vi "3color creation-cluster-2.vi"(4 "color":T1(array[cluster]) {"min" step=0.01 format="%_2f"; "max" step=0.1 format="%_3f"}, 5 "Array 4":bool[](array[boolean])=[TRUE, TRUE, TRUE], 7 "Array 3":dbl[][](array[numeric])=array90x160[14400 elements], 8 "Array 2":dbl[][](array[numeric])=array90x160[14400 elements], 9 "Array":dbl[][](array[numeric])=array90x160[14400 elements]) -> (0 "new picture":picture, 1 "ch3":picture, 2 "ch2":picture, 3 "ch1":picture)   [LabVIEW 2018]
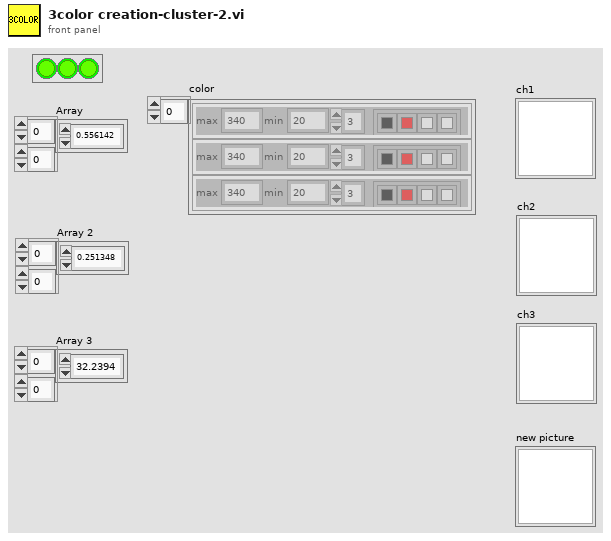
[diagram p1: front panel]
types:
  T1 = cluster{"color array":u32[], "num of colors":i32, "max":dbl, "min":dbl}[]
  T2 = cluster{"color array":u32[], "num of colors":i32, "max":dbl, "min":dbl}
  T3 = typedef "imagedata.ctl" = cluster{"image type":i32, "image depth":i32, "image":u8[], "mask":u8[], "colors":u32[], "Rectangle":cluster{"left":i16, "top":i16, "right":i16, "bottom":i16}}
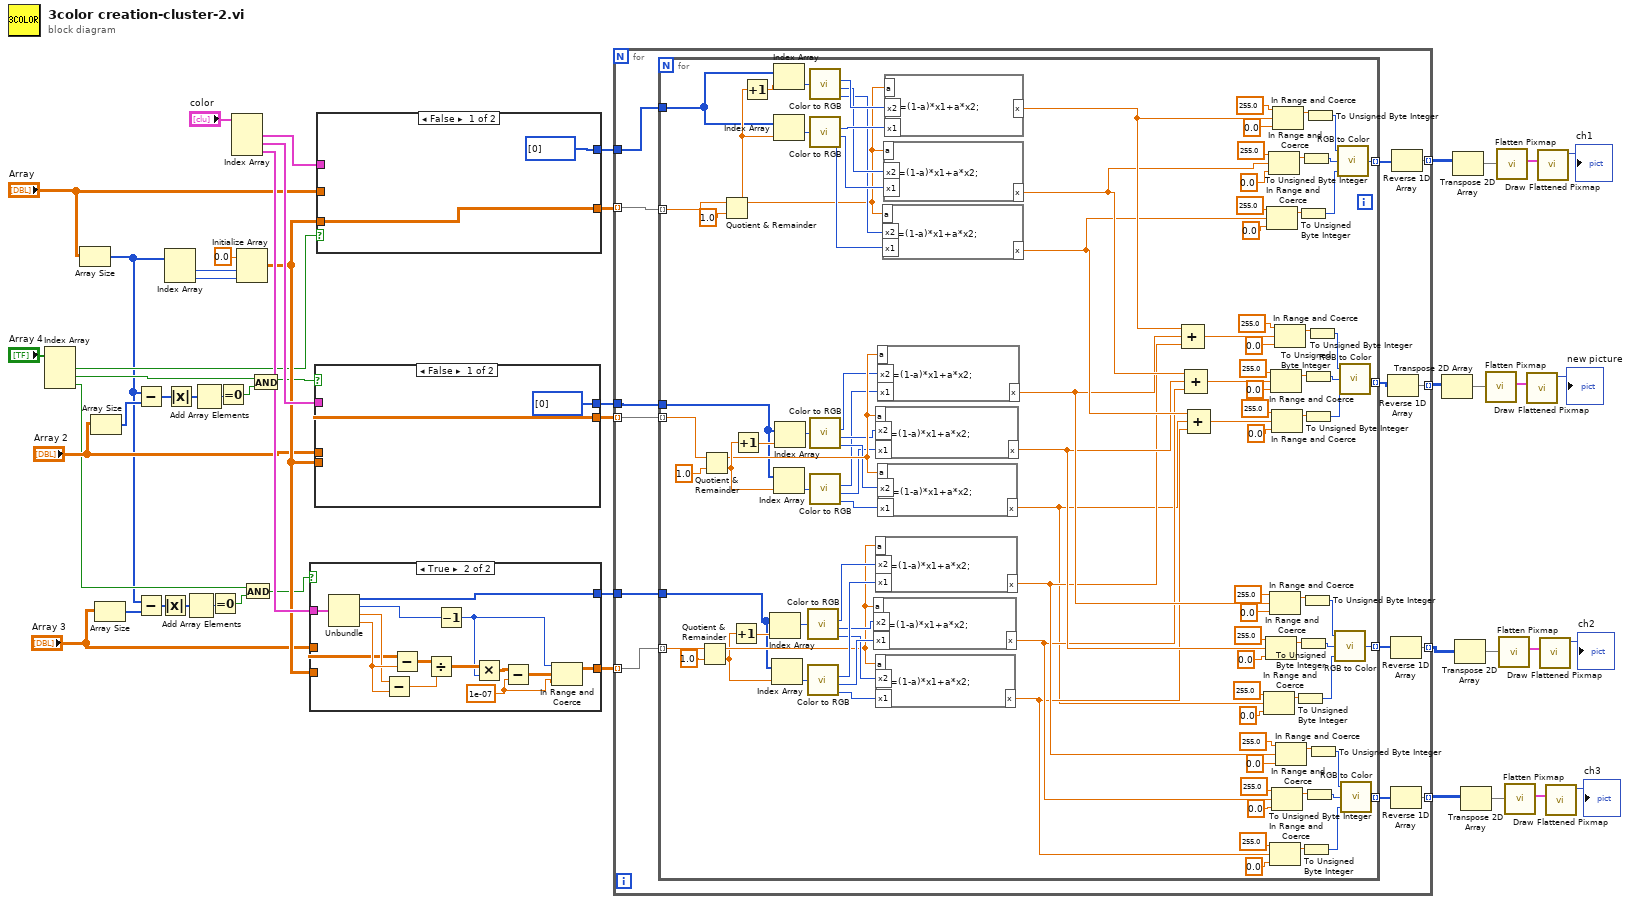
[diagram p0: block diagram]
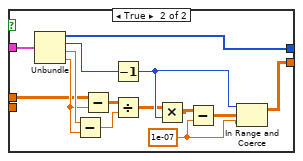
[diagram p2: hidden frame]
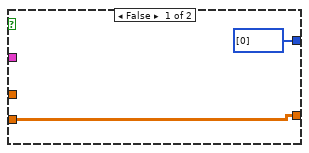
[diagram p3: hidden frame]
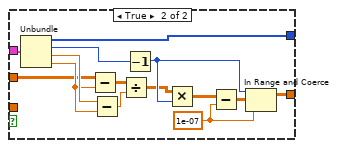
[diagram p4: hidden frame]
diagram:
  n1 = Index Array(array="Array 4") -> (element #1=w19:bool, element #2=w18:bool, element #3=w6:bool)  [unwired: 3 in]
  n2 = Array Size(array="Array") -> (size(s)=w4:i32[])
  n3 = Array Size(array="Array 2") -> (size(s)=w14:i32[])
  n4 = Array Size(array="Array 3") -> (size(s)=w7:i32[])
  n5 = Subtract(x=w4, y=w14) -> (x-y=w13:i32[])
  n6 = Subtract(x=w4, y=w7) -> (x-y=w8:i32[])
  n7 = Absolute Value(x=w8) -> (abs(x)=w2:i32[])
  n8 = Index Array(array=w4) -> (element #1=w22:i32, element #2=w23:i32)  [unwired: 2 in]
  n9 = Absolute Value(x=w13) -> (abs(x)=w1:i32[])
  n10 = Add Array Elements(numeric array=w2) -> (sum=w9:i32)
  n11 = Add Array Elements(numeric array=w1) -> (sum=w12:i32)
  n12 = Equal To 0?(x=w9) -> (x = 0?=w10:bool)
  n13 = Equal To 0?(x=w12) -> (x = 0?=w11:bool)
  n14 = Index Array(array="color") -> (element #1=w27:T2, element #2=w26:T2, element #3=w25:T2)  [unwired: 3 in]
  n15 = Initialize Array(0.0 ("element"), w22, w23) -> (w20:dbl[][])
  n16 = And(x=w6, y=w10) -> (x .and. y?=w5:bool)
  n17 = And(x=w18, y=w11) -> (x .and. y?=w15:bool)
  n18 = case shown="True" w5 {
    tunnel: [u32[] [0] ("color array") w56] -> w43
    tunnel: [w52 w55] -> w42
    tunnel: w25 -> [_ w54]
    tunnel: "Array 3" -> [_ w53]
    tunnel: w20 -> [w52 _]
    frame False {
    }
    frame True {
      w59 = 1e-07
      n19 = Unbundle(w54) -> ("color array"=w56:u32[], "num of colors"=w61:i32, "max"=w64:dbl, "min"=w65:dbl)
      n20 = Subtract(x=w64, y=w65) -> (x-y=w62:dbl)
      n21 = Subtract(x=w53, y=w65) -> (x-y=w63:dbl[][])
      n22 = Divide(x=w63, y=w62) -> (x/y=w66:dbl[][])
      n23 = Decrement(x=w61) -> (x-1=w57:i32)
      n24 = Multiply(x=w66, y=w57) -> (x*y=w58:dbl[][])
      n25 = Subtract(x=w58, y=w59) -> (x-y=w60:dbl[][])
      n26 = In Range and Coerce(upper limit=w57, x=w60, lower limit=w59) -> (coerced(x)=w55:dbl[][])  [unwired: 1 out]
    }
  }
  n27 = case shown="False" w15 {
    tunnel: [w68 w82] -> w50
    tunnel: [u32[] [0] ("color array") w81] -> w44
    tunnel: w26 -> [_ w80]
    tunnel: "Array 2" -> [_ w69]
    tunnel: w20 -> [w68 _]
    frame False {
    }
    frame True {
      w77 = 1e-07
      n28 = Unbundle(w80) -> ("color array"=w81:u32[], "num of colors"=w75:i32, "max"=w72:dbl, "min"=w71:dbl)
      n29 = Subtract(x=w72, y=w71) -> (x-y=w74:dbl)
      n30 = Subtract(x=w69, y=w71) -> (x-y=w73:dbl[][])
      n31 = Decrement(x=w75) -> (x-1=w79:i32)
      n32 = Divide(x=w73, y=w74) -> (x/y=w70:dbl[][])
      n33 = Multiply(x=w70, y=w79) -> (x*y=w78:dbl[][])
      n34 = Subtract(x=w78, y=w77) -> (x-y=w76:dbl[][])
      n35 = In Range and Coerce(upper limit=w79, x=w76, lower limit=w77) -> (coerced(x)=w82:dbl[][])  [unwired: 1 out]
    }
  }
  n36 = case shown="False" w19 {
    tunnel: [w84 w96] -> w48
    tunnel: [u32[] [0] ("color array") w93] -> w45
    tunnel: w27 -> [_ w86]
    tunnel: "Array" -> [_ w85]
    tunnel: w20 -> [w84 _]
    frame False {
    }
    frame True {
      w95 = 1e-07
      n37 = Unbundle(w86) -> ("color array"=w93:u32[], "num of colors"=w92:i32, "max"=w91:dbl, "min"=w90:dbl)
      n38 = Subtract(x=w85, y=w90) -> (x-y=w89:dbl[][])
      n39 = Subtract(x=w91, y=w90) -> (x-y=w88:dbl)
      n40 = Divide(x=w89, y=w88) -> (x/y=w87:dbl[][])
      n41 = Decrement(x=w92) -> (x-1=w98:i32)
      n42 = Multiply(x=w87, y=w98) -> (x*y=w97:dbl[][])
      n43 = Subtract(x=w97, y=w95) -> (x-y=w94:dbl[][])
      n44 = In Range and Coerce(upper limit=w98, x=w94, lower limit=w95) -> (coerced(x)=w96:dbl[][])  [unwired: 1 out]
    }
  }
  n45 = for {
    tunnel: w48 -> [w112] mode=indexing
    tunnel: w45 -> [w111]
    tunnel: w50 -> [w110] mode=indexing
    tunnel: [w107] -> w46 mode=indexing
    tunnel: w44 -> [w108]
    tunnel: w43 -> [w106]
    tunnel: w42 -> [w105] mode=indexing
    tunnel: [w103] -> w29 mode=indexing
    tunnel: [w101] -> w30 mode=indexing
    tunnel: [w99] -> w31 mode=indexing
    n46 = for {
      tunnel: w112 -> [w114] mode=indexing
      tunnel: w111 -> [w194]
      tunnel: w110 -> [w113] mode=indexing
      tunnel: [w193] -> w109 mode=indexing
      tunnel: w108 -> [w192]
      tunnel: w106 -> [w164]
      tunnel: w105 -> [w163] mode=indexing
      tunnel: [w124] -> w100 mode=indexing
      tunnel: [w123] -> w102 mode=indexing
      tunnel: [w122] -> w104 mode=indexing
      n47 = Quotient & Remainder(x=w163, y=1.0) -> (x-y*floor(x/y)=w166:dbl, floor(x/y)=w165:dbl)
      n48 = Quotient & Remainder(x=w113, y=1.0) -> (x-y*floor(x/y)=w205:dbl, floor(x/y)=w206:dbl)
      n49 = Quotient & Remainder(x=w114, y=1.0) -> (x-y*floor(x/y)=w208:dbl, floor(x/y)=w207:dbl)
      n50 = Increment(x=w165) -> (x+1=w175:dbl)
      n51 = Increment(x=w206) -> (x+1=w196:dbl)
      n52 = Increment(x=w207) -> (x+1=w217:dbl)
      n53 = Index Array(array=w164, index=w175) -> (element=w174:u32)
      n54 = Index Array(array=w164, index=w165) -> (element=w173:u32)
      n55 = Index Array(array=w194, index=w217) -> (element=w216:u32)
      n56 = Index Array(array=w194, index=w207) -> (element=w215:u32)
      n57 = Index Array(array=w192, index=w206) -> (element=w198:u32)
      n58 = Index Array(array=w192, index=w196) -> (element=w197:u32)
      n59 = call <vilib>:"Color to RGB.vi"("Color"=w174) -> ("R"=w171:u8, "G"=w169:u8, "B"=w167:u8)  [unwired: 1 out]
      n60 = call <vilib>:"Color to RGB.vi"("Color"=w173) -> ("R"=w172:u8, "G"=w170:u8, "B"=w168:u8)  [unwired: 1 out]
      n61 = call <vilib>:"Color to RGB.vi"("Color"=w216) -> ("R"=w213:u8, "G"=w211:u8, "B"=w209:u8)  [unwired: 1 out]
      n62 = call <vilib>:"Color to RGB.vi"("Color"=w215) -> ("R"=w214:u8, "G"=w212:u8, "B"=w210:u8)  [unwired: 1 out]
      n63 = call <vilib>:"Color to RGB.vi"("Color"=w197) -> ("R"=w200:u8, "G"=w202:u8, "B"=w204:u8)  [unwired: 1 out]
      n64 = call <vilib>:"Color to RGB.vi"("Color"=w198) -> ("R"=w199:u8, "G"=w201:u8, "B"=w203:u8)  [unwired: 1 out]
      n65 = formula code="x=(1-a)*x1+a*x2;"("a"=w166, "x2"=w169, "x1"=w170) -> ("x"=w126:dbl)
      n66 = formula code="x=(1-a)*x1+a*x2;"("a"=w205, "x2"=w202, "x1"=w201) -> ("x"=w128:dbl)
      n67 = formula code="x=(1-a)*x1+a*x2;"("a"=w166, "x2"=w171, "x1"=w172) -> ("x"=w127:dbl)
      n68 = formula code="x=(1-a)*x1+a*x2;"("a"=w166, "x2"=w167, "x1"=w168) -> ("x"=w125:dbl)
      n69 = formula code="x=(1-a)*x1+a*x2;"("a"=w205, "x2"=w200, "x1"=w199) -> ("x"=w129:dbl)
      n70 = formula code="x=(1-a)*x1+a*x2;"("a"=w205, "x2"=w204, "x1"=w203) -> ("x"=w115:dbl)
      n71 = formula code="x=(1-a)*x1+a*x2;"("a"=w208, "x2"=w209, "x1"=w210) -> ("x"=w148:dbl)
      n72 = formula code="x=(1-a)*x1+a*x2;"("a"=w208, "x2"=w211, "x1"=w212) -> ("x"=w149:dbl)
      n73 = formula code="x=(1-a)*x1+a*x2;"("a"=w208, "x2"=w213, "x1"=w214) -> ("x"=w150:dbl)
      n74 = Compound Arithmetic op=ADD(w150, w129, w127) -> (w177:dbl)
      n75 = Compound Arithmetic op=ADD(w149, w128, w126) -> (w178:dbl)
      n76 = Compound Arithmetic op=ADD(w148, w115, w125) -> (w179:dbl)
      n77 = In Range and Coerce(upper limit=255.0, x=w115, lower limit=0.0) -> (coerced(x)=w147:dbl)  [unwired: 1 out]
      n78 = In Range and Coerce(upper limit=255.0, x=w128, lower limit=0.0) -> (coerced(x)=w146:dbl)  [unwired: 1 out]
      n79 = In Range and Coerce(upper limit=255.0, x=w148, lower limit=0.0) -> (coerced(x)=w151:dbl)  [unwired: 1 out]
      n80 = In Range and Coerce(upper limit=255.0, x=w149, lower limit=0.0) -> (coerced(x)=w153:dbl)  [unwired: 1 out]
      n81 = In Range and Coerce(upper limit=255.0, x=w129, lower limit=0.0) -> (coerced(x)=w144:dbl)  [unwired: 1 out]
      n82 = In Range and Coerce(upper limit=255.0, x=w125, lower limit=0.0) -> (coerced(x)=w130:dbl)  [unwired: 1 out]
      n83 = In Range and Coerce(upper limit=255.0, x=w178, lower limit=0.0) -> (coerced(x)=w189:dbl)  [unwired: 1 out]
      n84 = In Range and Coerce(upper limit=255.0, x=w179, lower limit=0.0) -> (coerced(x)=w191:dbl)  [unwired: 1 out]
      n85 = In Range and Coerce(upper limit=255.0, x=w126, lower limit=0.0) -> (coerced(x)=w131:dbl)  [unwired: 1 out]
      n86 = In Range and Coerce(upper limit=255.0, x=w150, lower limit=0.0) -> (coerced(x)=w155:dbl)  [unwired: 1 out]
      n87 = In Range and Coerce(upper limit=255.0, x=w177, lower limit=0.0) -> (coerced(x)=w187:dbl)  [unwired: 1 out]
      n88 = In Range and Coerce(upper limit=255.0, x=w127, lower limit=0.0) -> (coerced(x)=w133:dbl)  [unwired: 1 out]
      n89 = To Unsigned Byte Integer(number=w147) -> (unsigned 8bit integer=w140:u8)
      n90 = To Unsigned Byte Integer(number=w151) -> (unsigned 8bit integer=w160:u8)
      n91 = To Unsigned Byte Integer(number=w146) -> (unsigned 8bit integer=w141:u8)
      n92 = To Unsigned Byte Integer(number=w153) -> (unsigned 8bit integer=w159:u8)
      n93 = To Unsigned Byte Integer(number=w130) -> (unsigned 8bit integer=w137:u8)
      n94 = To Unsigned Byte Integer(number=w144) -> (unsigned 8bit integer=w142:u8)
      n95 = To Unsigned Byte Integer(number=w189) -> (unsigned 8bit integer=w183:u8)
      n96 = To Unsigned Byte Integer(number=w191) -> (unsigned 8bit integer=w182:u8)
      n97 = To Unsigned Byte Integer(number=w131) -> (unsigned 8bit integer=w136:u8)
      n98 = To Unsigned Byte Integer(number=w155) -> (unsigned 8bit integer=w158:u8)
      n99 = To Unsigned Byte Integer(number=w187) -> (unsigned 8bit integer=w184:u8)
      n100 = To Unsigned Byte Integer(number=w133) -> (unsigned 8bit integer=w135:u8)
      n101 = call <vilib>:"RGB to Color.vi"("B"=w140, "G"=w141, "R"=w142) -> ("Color"=w123:u32)
      n102 = call <vilib>:"RGB to Color.vi"("B"=w160, "G"=w159, "R"=w158) -> ("Color"=w124:u32)
      n103 = call <vilib>:"RGB to Color.vi"("B"=w182, "G"=w183, "R"=w184) -> ("Color"=w193:u32)
      n104 = call <vilib>:"RGB to Color.vi"("B"=w137, "G"=w136, "R"=w135) -> ("Color"=w122:u32)
    }
    n105 = Reverse 1D Array(array=w109) -> (reversed array=w107:u32[])
    n106 = Reverse 1D Array(array=w102) -> (reversed array=w101:u32[])
    n107 = Reverse 1D Array(array=w104) -> (reversed array=w103:u32[])
    n108 = Reverse 1D Array(array=w100) -> (reversed array=w99:u32[])
  }
  n109 = Transpose 2D Array(2D array=w46) -> (transposed array=w49:u32[][])
  n110 = Transpose 2D Array(2D array=w31) -> (transposed array=w38:u32[][])
  n111 = Transpose 2D Array(2D array=w30) -> (transposed array=w37:u32[][])
  n112 = Transpose 2D Array(2D array=w29) -> (transposed array=w32:u32[][])
  n113 = call <vilib>:"Flatten Pixmap.vi"("24-bit pixmap"=w49) -> ("image data"=w47:T3)  [unwired: 10 in]
  n114 = call <vilib>:"Flatten Pixmap.vi"("24-bit pixmap"=w38) -> ("image data"=w39:T3)  [unwired: 10 in]
  n115 = call <vilib>:"Flatten Pixmap.vi"("24-bit pixmap"=w37) -> ("image data"=w36:T3)  [unwired: 10 in]
  n116 = call <vilib>:"Flatten Pixmap.vi"("24-bit pixmap"=w32) -> ("image data"=w33:T3)  [unwired: 10 in]
  n117 = call <vilib>:"Draw Flattened Pixmap.vi"("image data"=w47) -> ("new picture"=→"new picture":picture)  [unwired: 8 in]
  n118 = call <vilib>:"Draw Flattened Pixmap.vi"("image data"=w39) -> ("new picture"=→"ch1":picture)  [unwired: 8 in]
  n119 = call <vilib>:"Draw Flattened Pixmap.vi"("image data"=w36) -> ("new picture"=→"ch2":picture)  [unwired: 8 in]
  n120 = call <vilib>:"Draw Flattened Pixmap.vi"("image data"=w33) -> ("new picture"=→"ch3":picture)  [unwired: 8 in]
